vi "THzTime_SPEED_control_3_points_scan_TA_170301.vi"(1 "ESP300 Axis":i8=1, 2 "ESP300 Address":string="1", 4 "Lockin Address":string="12") -> ()   [LabVIEW 2010]
panel:
  out "Current Round":i32
  in  "ESP300 Axis 2":i8=1
  in  "Delay (ms)":u32
  in  "# of Round":i8=2
  in  "Position 3":sgl=-3.0 min=-75 max=75 format="%#.3f"
  in  "Position 2":sgl=-3.0 min=-75 max=75 format="%#.3f"
  in  "Position 1":sgl=-3.0 min=-75 max=75 format="%#.3f"
  out "Y position":dbl=-149.05 format="%#.3p"
  out "X position":dbl=857.9 format="%#.3p"
  out "Power meter":dbl=68.74000000000001 format="%#.3p"
  in  "Save File Name":string
  in  "Launch server?":bool
  in  "Authorize?":bool=TRUE
  in  "CONEX-PSD9 Instrument Key 2":string="CONEX-PSD (A6ULD43K)"
  in  "Interdelay (ms)":dbl
  in  "pre delay(ms)":dbl=10.0
  out "Lock-in Y-Channel":dbl=2.5466e-11 format="%#.3p"
  out "Lock-in X-Channel":dbl=-5.457e-12 format="%#.3p"
  out "THz Time-domain Signal Wave":cluster{"x-axis":sgl[], "y-axis":dbl[]}(graph)={"x-axis"=[-3.0, -2.99, -2.98, -2.97, -2.96, -2.95, -2.94, -2.93, -2.92, -2.91, -2.9, -2.89, -2.88, -2.87, -2.86, -2.85, -2.84, -2.83, -2.82, -2.81, -2.8, -2.79, -2.78, -2.77, -2.76, -2.75, -2.74, -2.73, -2.72, -2.71, -2.7, -2.69, -2.68, -2.67, -2.66, -2.65, -2.64, -2.63, -2.6200001, -2.61, -2.6, -2.59, -2.58, -2.57, -2.56, -2.55, -2.54, -2.53, -2.52, -2.51, -2.5, -2.49, -2.48, -2.47, -2.46, -2.45, -2.44, -2.43, -2.42, -2.41, -2.4, -2.39, -2.38, -2.3700001, -2.3600001, -2.35, -2.34, -2.33, -2.32, -2.31, -2.3, -2.29, -2.28, -2.27, -2.26, -2.25, -2.24, -2.23, -2.22, -2.21, -2.2, -2.19, -2.18, -2.17, -2.16, -2.15, -2.14, -2.13, -2.1200001, -2.1100001, -2.1, -2.09, -2.08, -2.07, -2.06, -2.05, -2.04, -2.03, -2.02, -2.01, -2.0, -1.99, -1.98, -1.97, -1.96, -1.95, -1.94, -1.9300001, -1.9200001, -1.91, -1.9, -1.89, -1.88, -1.87, -1.86, -1.85, -1.84, -1.83, -1.82, -1.8100001, -1.8000001, -1.7900001, -1.78, -1.77, -1.76, -1.75, -1.74, -1.73, -1.72, -1.71, -1.7, -1.69, -1.6800001, -1.6700001, -1.6600001, -1.65, -1.64, -1.63, -1.62, -1.61, -1.6, -1.59, -1.58, -1.57, -1.5600001, -1.5500001, -1.5400001, -1.5300001, -1.52, -1.51, -1.5, -1.49, -1.48, -1.47, -1.46, -1.45, -1.44, -1.4300001, -1.4200001, -1.4100001, -1.4000001, -1.39, -1.38, -1.37, -1.36, -1.35, -1.34, -1.33, -1.32, -1.3100001, -1.3000001, -1.2900001, -1.2800001, -1.27, -1.26, -1.25, -1.24, -1.23, -1.22, -1.21, -1.2, -1.19, -1.1800001, -1.1700001, -1.1600001, -1.1500001, -1.14, -1.13, -1.12, -1.11, -1.1, -1.09, -1.08, -1.07, -1.0600001, -1.0500001, -1.0400001, -1.0300001, -1.0200001, -1.01, -1.0, -0.99000007], "y-axis"=[6.18461e-11, 6.18461e-11, 6.275559999999999e-11, 6.457460000000001e-11, 6.54841e-11, 6.63936e-11, 6.821255e-11, 7.00315e-11, 7.18505e-11, 7.36695e-11, 7.54885e-11, 7.6398e-11, 7.6398e-11, 7.8217e-11, 7.8217e-11, 7.8217e-11, 7.8217e-11, 7.8217e-11, 7.8217e-11, 7.8217e-11, 7.8217e-11, 7.8217e-11, 7.8217e-11, 7.8217e-11, 7.73075e-11, 7.6398e-11, 7.54885e-11, 7.4579e-11, 7.4579e-11, 7.4579e-11, 7.4579e-11, 7.4579e-11, 7.4579e-11, 7.4579e-11, 7.36695e-11, 7.276e-11, 7.276e-11, 7.276e-11, 7.18505e-11, 7.18505e-11, 7.276e-11, 7.18505e-11, 7.0941e-11, 7.0941e-11, 7.00315e-11, 6.9122e-11, 6.821255e-11, 6.63936e-11, 6.457460000000001e-11, 6.275559999999999e-11, 6.18461e-11, 6.18461e-11, 6.275559999999999e-11, 6.36651e-11, 6.63936e-11, 6.912205e-11, 7.275999999999999e-11, 7.6398e-11, 7.91265e-11, 8.09455e-11, 8.27645e-11, 8.3674e-11, 8.3674e-11, 8.3674e-11, 8.27645e-11, 8.09455e-11, 7.821699999999999e-11, 7.36695e-11, 6.821255e-11, 6.09366e-11, 5.54795e-11, 4.911295e-11, 4.2746500000000003e-11, 3.7289500000000003e-11, 3.2742e-11, 3.001355e-11, 2.7285e-11, 2.7285e-11, 2.819455e-11, 3.092305e-11, 3.4561000000000003e-11, 3.7289500000000003e-11, 3.9108499999999995e-11, 4.09275e-11, 4.45655e-11, 4.638445e-11, 5.00224e-11, 5.18414e-11, 5.36604e-11, 5.72985e-11, 5.82081e-11, 5.82081e-11, 5.82081e-11, 6.00271e-11, 6.09366e-11, 6.275559999999999e-11, 6.457460000000001e-11, 6.730305e-11, 7.00315e-11, 7.18505e-11, 7.36695e-11, 7.54885e-11, 7.6398e-11, 7.73075e-11, 7.8217e-11, 7.8217e-11, 7.8217e-11, 7.8217e-11, 7.8217e-11, 7.8217e-11, 7.8217e-11, 7.8217e-11, 7.8217e-11, 7.8217e-11, 7.8217e-11, 7.8217e-11, 7.91265e-11, 8.0036e-11, 8.0036e-11, 7.91265e-11, 7.8217e-11, 7.8217e-11, 7.8217e-11, 7.8217e-11, 7.91265e-11, 8.0036e-11, 8.0036e-11, 8.0036e-11, 8.09455e-11, 8.1855e-11, 8.09455e-11, 8.0036e-11, 7.91265e-11, 7.8217e-11, 7.8217e-11, 7.73075e-11, 7.54885e-11, 7.36695e-11, 7.18505e-11, 6.9122e-11, 6.73031e-11, 6.54841e-11, 6.457460000000001e-11, 6.36651e-11, 6.275559999999999e-11, 6.09366e-11, 6.00271e-11, 6.00271e-11, 6.00271e-11, 6.00271e-11, 6.09366e-11, 6.18461e-11, 6.18461e-11, 6.18461e-11, 6.275559999999999e-11, 6.36651e-11, 6.457460000000001e-11, 6.54841e-11, 6.457460000000001e-11, 6.36651e-11, 6.36651e-11, 6.36651e-11, 6.36651e-11, 6.36651e-11, 6.36651e-11, 6.36651e-11, 6.36651e-11, 6.36651e-11, 6.36651e-11, 6.36651e-11, 6.36651e-11, 6.36651e-11, 6.457460000000001e-11, 6.54841e-11, 6.457460000000001e-11, 6.457460000000001e-11, 6.54841e-11, 6.63936e-11, 6.73031e-11, 6.73031e-11, 6.9122e-11, 6.73031e-11, 6.821255e-11, 6.9122e-11, 6.9122e-11, 6.73031e-11, 6.821255e-11, 6.9122e-11, 6.9122e-11, 6.9122e-11, 6.9122e-11, 6.821255e-11, 6.73031e-11, 6.73031e-11, 6.73031e-11, 6.73031e-11, 6.73031e-11, 6.73031e-11, 6.63936e-11, 6.63936e-11, 6.54841e-11, 6.54841e-11]}
  in  "Autosave Directory for Long-term Average Scan":path=path "D:/KHA/20140828_reference/20140829/MAX1"
  in  "OK Button":bool
  out "Data Type":string="outp ? 1"
  in  "Enum":enum16{"X", "Y", "Abs"}(ring)
  in  "Draw":bool
  in  "Exit Program":bool
  in  "Short term \nAverage#":i8=2
  in  "Step":sgl=0.01 min=0 max=10000 format="%.3f"
  in  "End Position":sgl=-1.0 min=-75 max=75 format="%#.3f"
  in  "Start Position":sgl=-3.0 min=-75 max=75 format="%#.3f"
  # "THz Experiment"
  # "Data"
  # "Auto-offset"
  # "Start Position (mm)"
  # "End Position (mm)"
  # "Step (mm)"
  # "Point Avg"
  # "Number of Round"
  # "Position 1 (mm)"
  # "Position 2 (mm)"
  # "Position 3 (mm)"
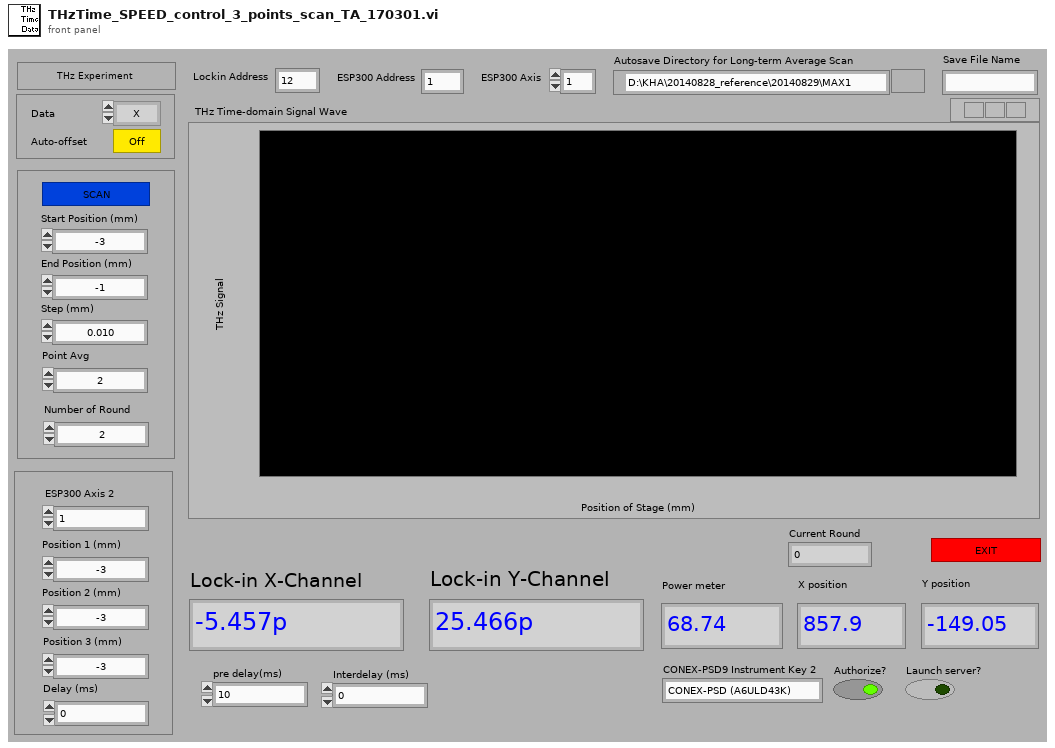
[diagram p1: front panel]
types:
  T1 = cluster{"ConexPSD Reference":refnum<k24>, "error out":errorcluster, "Component ID":i32}
  T2 = cluster{"Step Number":i32, "Step":sgl, "Start Position":sgl, "Time-out":i32, "Lockin Address":string, "Short term \nAverage#":i8, i32, "ESP300 Axis":i8, "Value":string, "pre delay(ms)":dbl, "Interdelay (ms)":dbl, "Autosave Directory for Long-term Average Scan":path, cluster{"ConexPSD Reference":refnum<k24>, "error out":errorcluster, "Component ID":i32}}
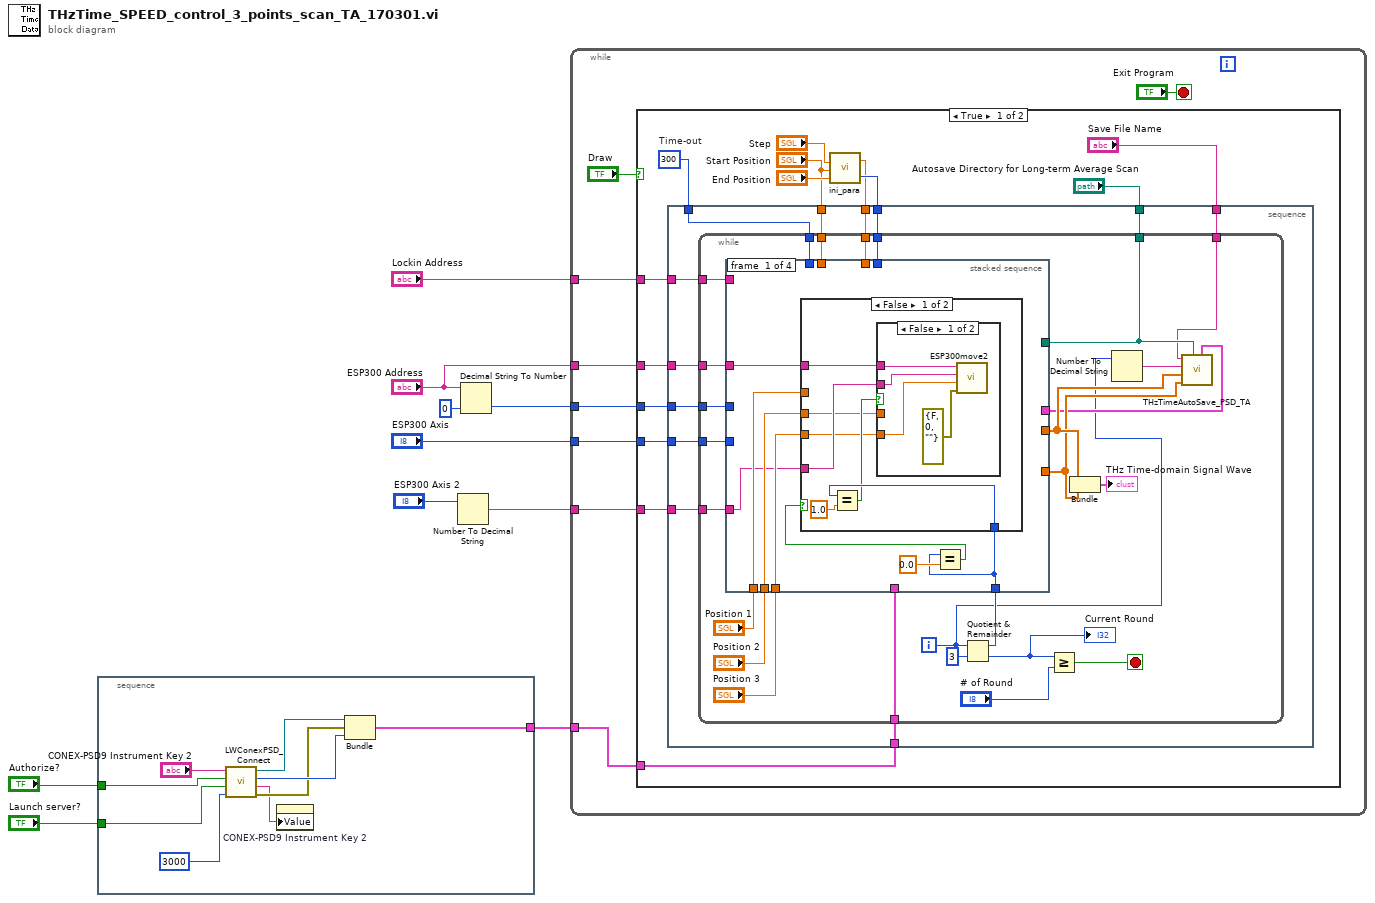
[diagram p0: block diagram]
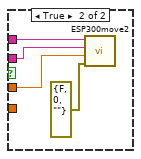
[diagram p2: hidden frame]
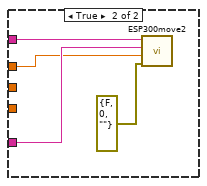
[diagram p3: hidden frame]
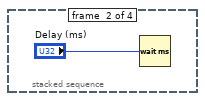
[diagram p4: hidden frame]
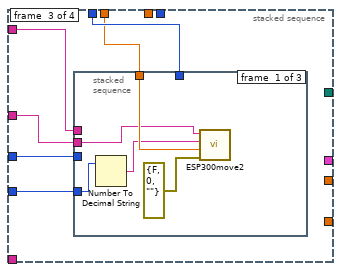
[diagram p5: hidden frame]
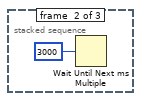
[diagram p6: hidden frame]
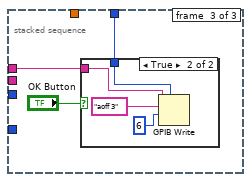
[diagram p7: hidden frame]
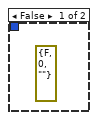
[diagram p8: hidden frame]
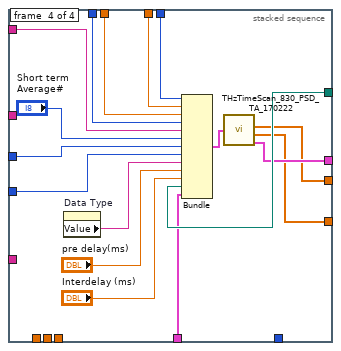
[diagram p9: hidden frame]
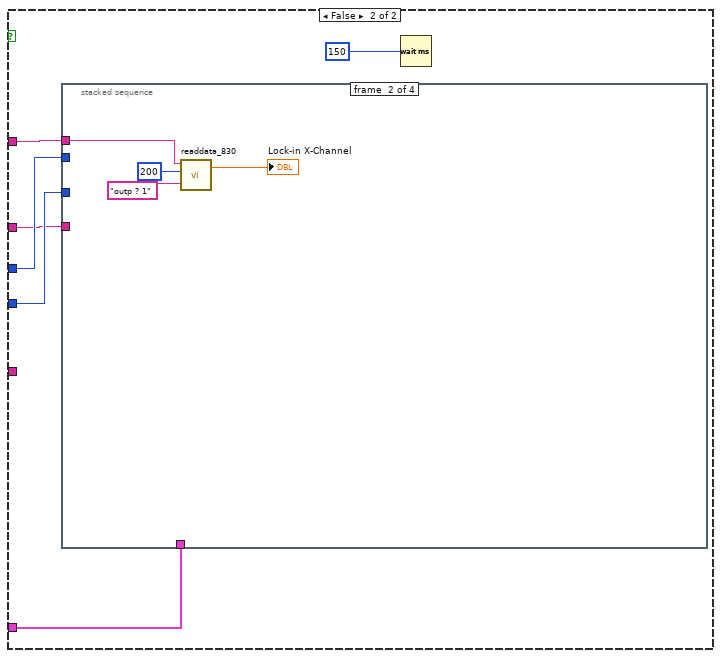
[diagram p10: hidden frame]
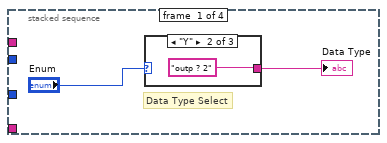
[diagram p11: hidden frame]
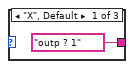
[diagram p12: hidden frame]
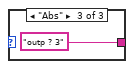
[diagram p13: hidden frame]
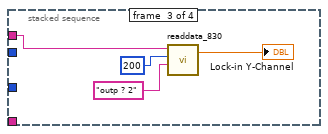
[diagram p14: hidden frame]
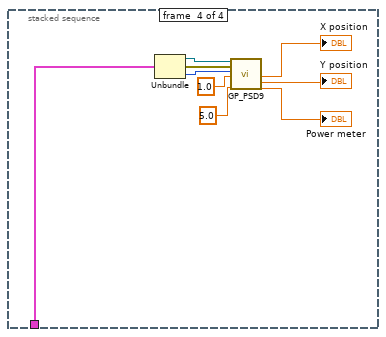
[diagram p15: hidden frame]
diagram:
  n1 = stacked-sequence {
    tunnel: "Authorize?" -> [w13]
    tunnel: [w12] -> w3
    tunnel: "Launch server?" -> [w11]
    frame #0 {
      n2 = call "LWConexPSD_Connect.vi"("DiscoverTimeout (10000 msec)"=3000, "Launch server? (True)"=w11, "Authorize? (True)"=w13, "Instrument Key"="CONEX-PSD9 Instrument Key 2") -> ("error out"=w17:errorcluster, "Instrument Key out"=w15:string, "Component ID"=w18:i32, "ConexPSD Reference"=w16:refnum<k24>)
      n3 = property on="CONEX-PSD9 Instrument Key 2" class="Str"("Value"=w15) -> ()  [unwired: 2 in, 2 out]
      n4 = Bundle("ConexPSD Reference"=w16, "error out"=w17, "Component ID"=w18) -> (w12:T1)  [unwired: 1 in]
    }
  }
  n5 = Number To Decimal String(number="ESP300 Axis 2") -> (decimal integer string=w1:string)  [unwired: 1 in]
  n6 = Decimal String To Number(string="ESP300 Address", default (0L)=0 ("default (0 I32)")) -> (number=w8:i32)  [unwired: 1 in, 1 out]
  n7 = while {
    tunnel: "ESP300 Axis" -> [w25]
    tunnel: "Lockin Address" -> [w24]
    tunnel: w8 -> [w23]
    tunnel: "ESP300 Address" -> [w22]
    tunnel: w3 -> [w21]
    tunnel: w1 -> [w20]
    stop <- "Exit Program" stop-if-true
    n8 = case shown="True" "Draw" {
      tunnel: w24 -> [w41 w147]
      tunnel: w25 -> [w40 w149]
      tunnel: w23 -> [w39 w148]
      tunnel: w22 -> [w31 w145]
      tunnel: w21 -> [w30 w144]
      tunnel: w20 -> [w28 _]
      frame True {
        w38 = 300  # Time-out
        n9 = call "ini_para.vi"("End Position"="End Position", "Start Position"="Start Position", "Step"="Step") -> ("Step Number"=w35:i32, "Step"=w34:sgl)
        n10 = stacked-sequence {
          tunnel: w41 -> [w53]
          tunnel: w38 -> [w52]
          tunnel: w40 -> [w51]
          tunnel: w39 -> [w50]
          tunnel: w35 -> [w48]
          tunnel: w34 -> [w46]
          tunnel: "Start Position" -> [w49]
          tunnel: "Autosave Directory for Long-term Average Scan" -> [w47]
          tunnel: w31 -> [w45]
          tunnel: w30 -> [w44]
          tunnel: "Save File Name" -> [w43]
          tunnel: w28 -> [w42]
          frame #0 {
            n11 = while {
              tunnel: w53 -> [w79]
              tunnel: w52 -> [w78]
              tunnel: w51 -> [w77]
              tunnel: w50 -> [w76]
              tunnel: w49 -> [w75]
              tunnel: w48 -> [w74]
              tunnel: w47 -> [w73]
              tunnel: w46 -> [w72]
              tunnel: w45 -> [w70]
              tunnel: w44 -> [w69]
              tunnel: w43 -> [w68]
              tunnel: w42 -> [w58]
              i -> [w54]
              stop <- w55 stop-if-true
              n12 = Quotient & Remainder(x=w54, y=3) -> (x-y*floor(x/y)=w62:i32, floor(x/y)=w56:i32)
              "Current Round" <- w56
              n13 = stacked-sequence {
                tunnel: w79 -> [_ _ w113 w139]
                tunnel: w78 -> [_ _ w112 w140]
                tunnel: w77 -> [_ _ w111 w136]
                tunnel: w76 -> [_ _ w110 w137]
                tunnel: w75 -> [_ _ w109 w141]
                tunnel: w72 -> [_ _ _ w142]
                tunnel: w74 -> [_ _ _ w143]
                tunnel: [_ _ _ w127] -> w71
                tunnel: [_ _ _ w128] -> w65
                tunnel: w70 -> [w82 _ w108 _]
                tunnel: w73 -> [_ _ _ w132]
                tunnel: w69 -> [_ _ _ w131]
                tunnel: [_ _ _ w129] -> w64
                tunnel: w62 -> [w80 _ _ _]
                tunnel: "Position 1" -> [w85 _ _ _]
                tunnel: "Position 2" -> [w84 _ _ _]
                tunnel: "Position 3" -> [w83 _ _ _]
                tunnel: w58 -> [w81 _ _ _]
                frame #0 {
                  n14 = Equal?(x=w80, y=0.0) -> (x = y?=w86:bool)
                  n15 = case shown="False" w86 {
                    tunnel: w85 -> [_ w103]
                    tunnel: w84 -> [w89 _]
                    tunnel: w83 -> [w88 _]
                    tunnel: w82 -> [w91 w106]
                    tunnel: w81 -> [w90 w105]
                    tunnel: w80 -> [w93 _]
                    frame False {
                      n16 = Equal?(x=w93, y=1.0) -> (x = y?=w92:bool)
                      n17 = case shown="False" w92 {
                        tunnel: w91 -> [w97 w101]
                        tunnel: w90 -> [w96 w100]
                        tunnel: w89 -> [_ w99]
                        tunnel: w88 -> [w95 _]
                        frame False {
                          n18 = call "ESP300move2.vi"("ESP300 Address"=w97, "ESP300 Channel"=w96, "Target"=w95, "error in (no error) 2"=errorcluster {"status"=FALSE, "code"=0, "source"=""}) -> ()  [unwired: 6 in, 1 out]
                        }
                        frame True {
                          n19 = call "ESP300move2.vi"("ESP300 Address"=w101, "ESP300 Channel"=w100, "Target"=w99, "error in (no error) 2"=errorcluster {"status"=FALSE, "code"=0, "source"=""}) -> ()  [unwired: 6 in, 1 out]
                        }
                      }
                    }
                    frame True {
                      n20 = call "ESP300move2.vi"("ESP300 Address"=w106, "ESP300 Channel"=w105, "Target"=w103, "error in (no error) 2"=errorcluster {"status"=FALSE, "code"=0, "source"=""}) -> ()  [unwired: 6 in, 1 out]
                    }
                  }
                }
                frame #1 {
                  n21 = Wait (ms)(milliseconds to wait="Delay (ms)") -> ()  [unwired: 1 out]
                }
                frame #2 {
                  n22 = stacked-sequence {
                    tunnel: w113 -> [_ _ w121]
                    tunnel: w112 -> [_ _ w120]
                    tunnel: w111 -> [w115 _ _]
                    tunnel: w110 -> [_ _ _]
                    tunnel: w109 -> [w118 _ _]
                    tunnel: w108 -> [w116 _ _]
                    frame #0 {
                      n23 = Number To Decimal String(number=w115) -> (decimal integer string=w114:string)  [unwired: 1 in]
                      n24 = call "ESP300move2.vi"("ESP300 Address"=w116, "ESP300 Channel"=w114, "Target"=w118, "error in (no error) 2"=errorcluster {"status"=FALSE, "code"=0, "source"=""}) -> ()  [unwired: 6 in, 1 out]
                    }
                    frame #1 {
                      n25 = Wait Until Next ms Multiple(millisecond multiple=3000) -> ()  [unwired: 1 out]
                    }
                    frame #2 {
                      n26 = case shown="True" "OK Button" {
                        tunnel: w121 -> [_ w126]
                        tunnel: w120 -> [_ w124]
                        frame False {
                          (unwired) errorcluster {"status"=FALSE, "code"=0, "source"=""} ("error in")
                        }
                        frame True {
                          n27 = GPIB Write(0:w126, 1:"aoff 3" ("data"), 2:i16 6 ("mode (0)"), 4:w124) -> ()  [unwired: 1 in, 2 out]
                        }
                      }
                    }
                  }
                }
                frame #3 {
                  n28 = property on="Data Type" class="Str"() -> ("Value"=w135:string)  [unwired: 2 in, 2 out]
                  n29 = Bundle("Step Number"=w143, "Step"=w142, "Start Position"=w141, "Time-out"=w140, "Lockin Address"=w139, "Short term \nAverage#"="Short term \nAverage#", w137, "ESP300 Axis"=w136, "Value"=w135, "pre delay(ms)"="pre delay(ms)", "Interdelay (ms)"="Interdelay (ms)", "Autosave Directory for Long-term Average Scan"=w132, w131) -> (w130:T2)  [unwired: 1 in]
                  n30 = call "THzTimeScan_830_PSD_TA_170222.vi"("input"=w130) -> ("x-axis"=w127:sgl[], "y-axis"=w128:dbl[], "ext. out"=w129:cluster{dbl[], dbl[], dbl[], dbl[], string[]})  [unwired: 1 out]
                }
              }
              n31 = Greater Or Equal?(x=w56, y="# of Round") -> (x >= y?=w55:bool)
              n32 = Bundle("x-axis"=w71, "y-axis"=w65) -> (→"THz Time-domain Signal Wave":cluster{"x-axis":sgl[], "y-axis":dbl[]})  [unwired: 1 in]
              n33 = Number To Decimal String(number=w54) -> (decimal integer string=w66:string)  [unwired: 1 in]
              n34 = call "THzTimeAutoSave_PSD_TA.vi"("ext. out"=w64, "Autosave Directory for Long-term Average Scan"=w73, "y-axis"=w65, "x-axis"=w71, "String"=w66, "SaveFile name"=w68) -> ()  [unwired: 4 in]
            }
          }
        }
      }
      frame False {
        n35 = stacked-sequence {
          tunnel: w149 -> [_ _ _ _]
          tunnel: w148 -> [_ _ _ _]
          tunnel: w147 -> [_ w158 w162 _]
          tunnel: w145 -> [_ _ _ _]
          tunnel: w144 -> [_ _ _ w163]
          frame #0 {
            # "Data Type Select"
            n36 = case shown="\"Y\"" "Enum" {
              tunnel: ["outp ? 1" "outp ? 2" "outp ? 3"] -> w151
              frame "X", Default {
              }
              frame "Y" {
              }
              frame "Abs" {
              }
            }
            "Data Type" <- w151
          }
          frame #1 {
            n37 = call "readdata_830.vi"("Command"="outp ? 1", "timeout"=200, "Lockin Address"=w158) -> ("Data"=→"Lock-in X-Channel":dbl)  [unwired: 1 in, 1 out]
          }
          frame #2 {
            n38 = call "readdata_830.vi"("Command"="outp ? 2", "timeout"=200, "Lockin Address"=w162) -> ("Data"=→"Lock-in Y-Channel":dbl)  [unwired: 1 in, 1 out]
          }
          frame #3 {
            n39 = Unbundle(w163) -> ("ConexPSD Reference"=w171:refnum<k24>, "error out"=w170:errorcluster, "Component ID"=w169:i32)
            n40 = call "GP_PSD9.vi"("ConexPSD Reference"=w171, "error out"=w170, "Component ID"=w169, "Adress"=1.0 ("shot average"), "shot average"=5.0) -> ("PositionX"=→"X position":dbl, "PositionY"=→"Y position":dbl, "LaserPower"=→"Power meter":dbl)  [unwired: 8 in, 4 out]
          }
        }
        n41 = Wait (ms)(milliseconds to wait=u32 150) -> ()  [unwired: 1 out]
      }
    }
  }
